vi "Unflatten Value.vi"(8 "error in (no error)":errorcluster, 10 "Value":string, 11 "Boolean in":refnum<class "U32 1D.lvclass">) -> (0 "error out":errorcluster, 3 "Boolean out":refnum<class "U32 1D.lvclass">)   [LabVIEW 2020, in "U32 1D.lvclass"]
uses:
  <vilib>/gpm_packages/@cs/data-type-serializer/source/U32 1D/U32 1D.lvclass
  <vilib>/gpm_packages/@cs/data-type-serializer/source/U32 1D/U32 1D.lvclass/U32 1D.ctl
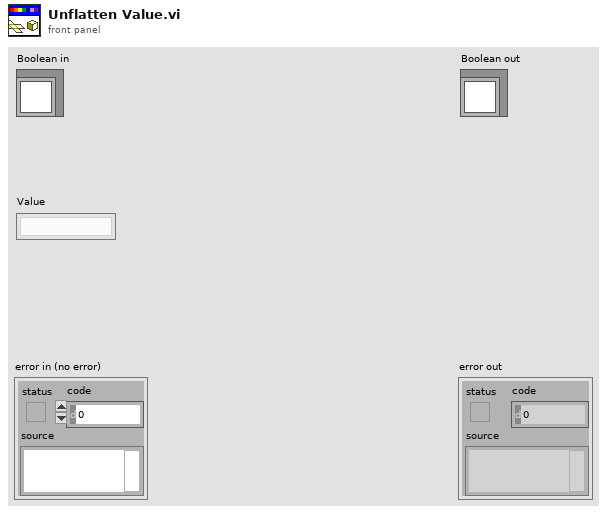
[diagram p1: front panel]
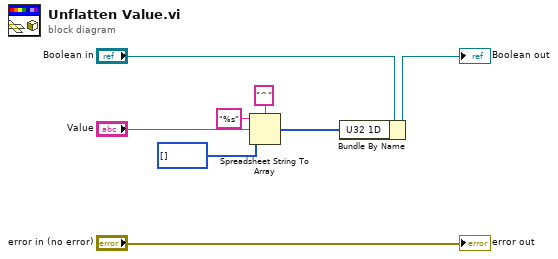
[diagram p0: block diagram]
diagram:
  n1 = Spreadsheet String To Array(delimiter (Tab)="^", format string="%s", spreadsheet string="Value", array type (2D Dbl)=u32[] [] ("Double 1D")) -> (array=w1:u32[])
  n2 = Bundle By Name(cluster="Boolean in", "U32 1D"=w1) -> (→"Boolean out":refnum<class "U32 1D.lvclass">)
  "error out" <- "error in (no error)"
